vi "get_mechanisms.vi"() -> (2 "Mechanisms":string[](array[string]))   [LabVIEW 2018]
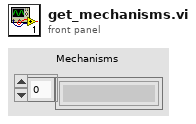
[diagram p1: front panel]
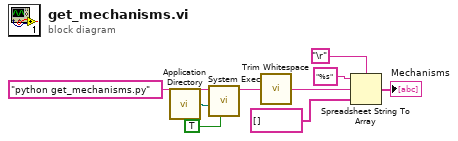
[diagram p0: block diagram]
diagram:
  n1 = call <vilib>:"Application Directory.vi"() -> ("Application Directory"=w8:path)
  n2 = call <vilib>:"System Exec.vi"("run minimized? (F)"=TRUE, "working directory"=w8, "command line"="python get_mechanisms.py") -> ("standard output"=w4:string)  [unwired: 5 in, 3 out]
  n3 = call <vilib>:"Trim Whitespace.vi"("string"=w4) -> ("trimmed string"=w3:string)  [unwired: 1 in]
  n4 = Spreadsheet String To Array(delimiter (Tab)="\r", format string="%s", spreadsheet string=w3, array type (2D Dbl)=string[] []) -> (array=→"Mechanisms":string[])
